vi "FTW-System-CommandLineExecute.vi"(0 "Command":string, 5 "Standard Input":string, 7 "Working Directory":path, 9 "Blocking?":bool=TRUE, 11 "error in":errorcluster) -> (4 "Standard Output":string, 6 "Standard Error":string, 8 "Return Code":i32, 15 "error out":errorcluster)   [LabVIEW 2013]
panel:
  # "Inputs"
  # "Outputs"
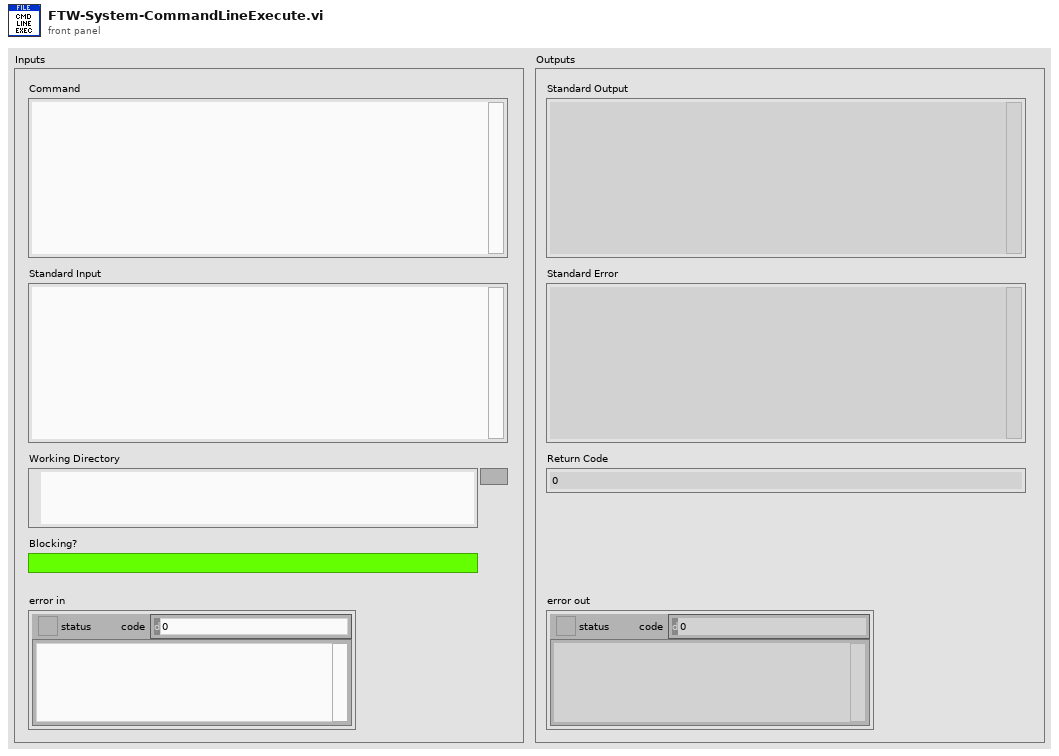
[diagram p1: front panel]
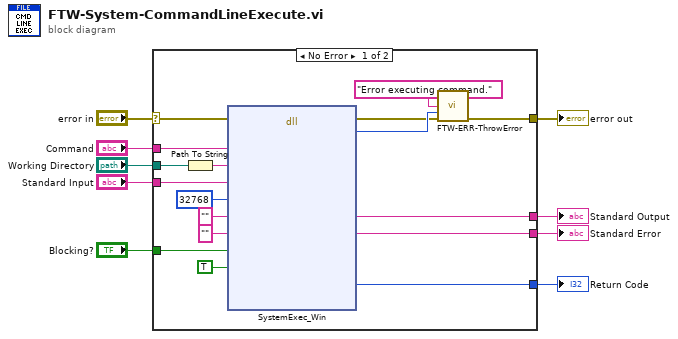
[diagram p0: block diagram]
diagram:
  n1 = case shown="No Error" "error in" {
    selector: "error in" -> [w26 w27]
    tunnel: "Working Directory" -> [w19 _]
    tunnel: [w20 w27] -> w7
    tunnel: "Standard Input" -> [w18 _]
    tunnel: "Command" -> [w17 _]
    tunnel: [w16 _] -> w4
    tunnel: [w15 _] -> w3
    tunnel: [w13 _] -> w2
    tunnel: "Blocking?" -> [w10 _]
    frame No Error {
      n2 = Path To String(path=w19) -> (string=w24:string)
      n3 = dll-call lib="LabVIEW" fn="SystemExec_Win"(error in=w26, "Command"=w17, "Working Directory"=w24, "Standard Input"=w18, "Expected Output Size"=u32 32768, "Standard Output"="", "Standard Error"="", "Blocking?"=w10, "Run Minimized"=TRUE) -> (error out=w21:errorcluster, "Return"=w23:i32, "Standard Output"=w16:string, "Standard Error"=w15:string, "Return Code"=w13:i32)  [unwired: 11 in, 1 out]
      n4 = call "FTW-ERR-ThrowError.vi"("Error Message"="Error executing command.", "Error Code"=w23, "error in"=w21) -> ("error out"=w20:errorcluster)  [unwired: 12 in]
    }
    frame Error {
    }
  }
  "error out" <- w7
  "Standard Output" <- w4
  "Standard Error" <- w3
  "Return Code" <- w2
